vi "Create Server SMO.vi"(8 "error in (no error)":errorcluster, 11 "RemoteControl in":refnum<class "RemoteControl.lvclass">) -> (0 "error out":errorcluster, 3 "RemoteControl out":refnum<class "RemoteControl.lvclass">)   [LabVIEW 2019, in "RemoteControl.lvclass"]
uses:
  RemoteControl.lvclass
  C:/Program Files (x86)/National Instruments/LabVIEW 2019/vi.lib/JKI/JKI SMO/SMO/SMO.lvclass
  Typedefs/RC Process Type--Enum.ctl
  RemoteControl.lvclass/RemoteControl.ctl
  <vilib>/JKI/JKI SMO/SMO/Typedefs/Public Events.ctl
  <vilib>/JKI/JKI SMO/SMO/Typedefs/SMOState --Enum.ctl
  <vilib>/JKI/JKI SMO/SMO/Typedefs/Reserve State--Enum.ctl
  Typedefs/PublicEvents--Cluster.ctl
  Typedefs/PublicEvents--RemoteControl.SendMessageFromProcess.ctl
  Typedefs/Message--Cluster.ctl
  <vilib>/JKI/JKI SMO/SMO/SMO.lvclass
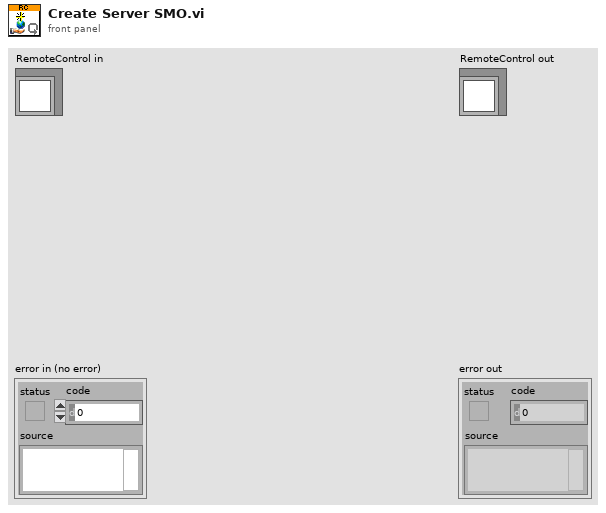
[diagram p1: front panel]
types:
  T1 = typedef "RemoteControl.lvclass/RC Process Type--Enum.ctl" = enum16{"Listener", "Server", "Client"}
  T2 = typedef "RemoteControl.lvclass/PublicEvents--Cluster.ctl" = cluster{"SendMessageFromProcess":refnum<user-event>}
  T3 = typedef "SMO.lvclass/Public Events.ctl" = cluster{"Error":refnum<user-event>, "State":refnum<user-event>, "Reserve State":refnum<user-event>}
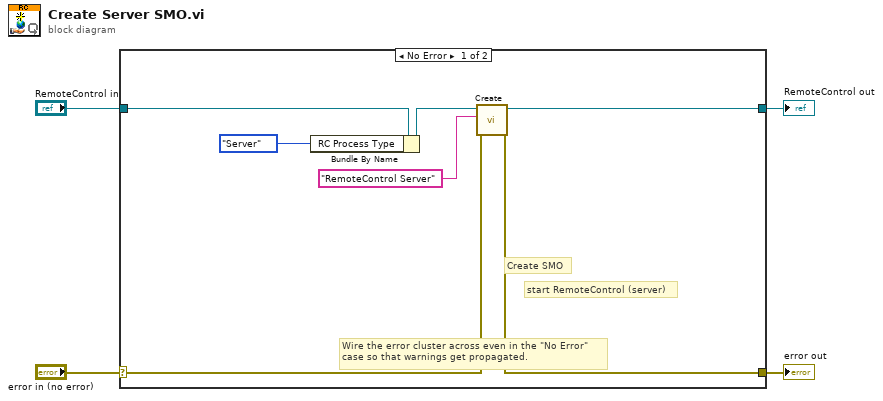
[diagram p0: block diagram]
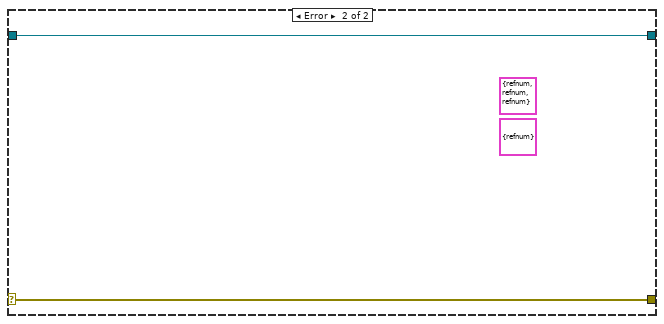
[diagram p2: hidden frame]
diagram:
  n1 = case shown="No Error" "error in (no error)" {
    selector: "error in (no error)" -> [w9 w13]
    tunnel: [w8 w13] -> w3
    tunnel: [w10 w12] -> w1
    tunnel: "RemoteControl in" -> [w11 w12]
    frame No Error {
      # "start RemoteControl (server)"
      # "Create SMO"
      # "Wire the error cluster across even in the \"No Error\"\ncase so that warnings get propagated."
      n2 = Bundle By Name(cluster=w11, "RC Process Type"=RC_Process_Type--Enum."Server") -> (w6:refnum<class "RemoteControl.lvclass">)
      n3 = call <vilib>:"Create.vi"("error in (no error)"=w9, "Subsystem Name (optional)"="RemoteControl Server" ("format string"), "SMO"=w6) -> ("error out"=w8:errorcluster, "SMO out"=w10:refnum<class "RemoteControl.lvclass">)  [unwired: 6 in, 1 out]
    }
    frame Error {
      (unwired) T2 {"SendMessageFromProcess"=refnum} ("RC Public Events")
      (unwired) T3 {"Error"=refnum, "State"=refnum, "Reserve State"=refnum} ("Public Events")
    }
  }
  "error out" <- w3
  "RemoteControl out" <- w1
